vi "Wizard_Msg.vi"(0 "Application_Directory":path, 11 "Error_In":errorcluster) -> (15 "Error_Out":errorcluster)   [LabVIEW 2023]
doc: "This is a VI work as one of the front panel of the Game, showing the message of wizard."
uses:
  Controls/Bool_Button.ctl
  Controls/State.ctl
panel:
  in  "Back?":T1
  in  "Next":T1
  out "Wizard_Msg":string
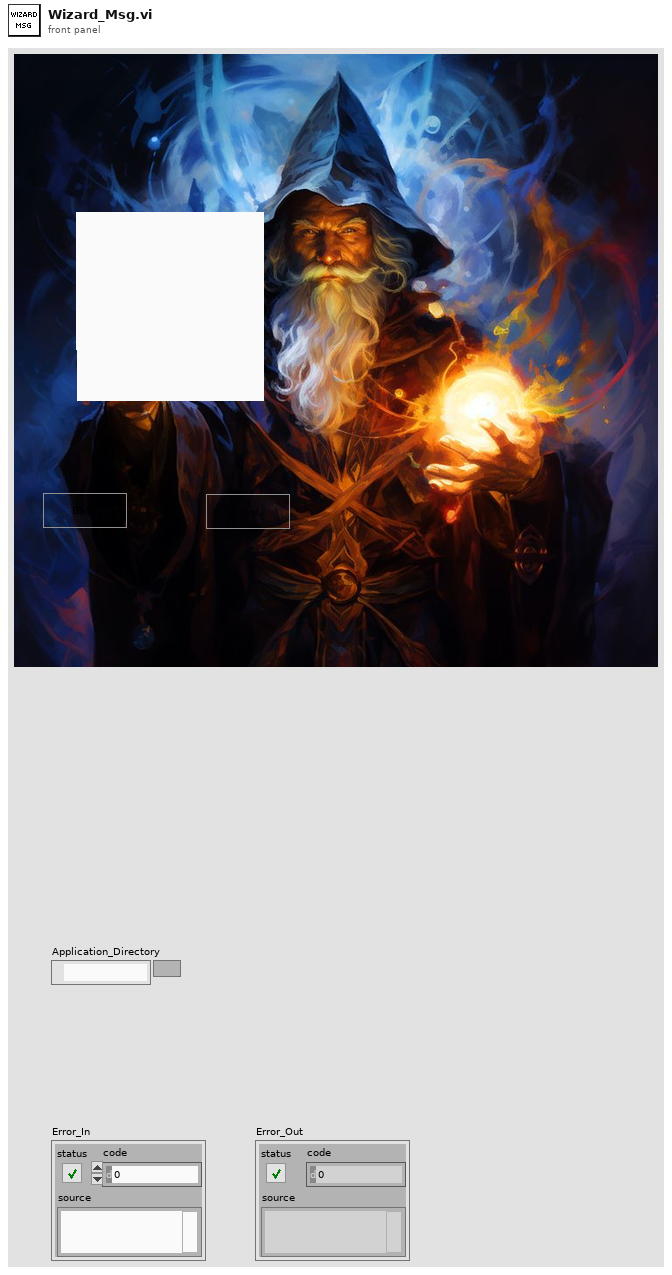
[diagram p1: front panel]
types:
  T1 = typedef "Bool_Button.ctl" = bool
  T2 = enum32{"Invalid", "Standard", "Closed", "Hidden", "Minimized", "Maximized"}
  T3 = typedef "State.ctl" = enum16{"Close", "Password_Popup", "Start_Popup", "Wizard_Msg", "Get_Name_DoB", "Lucky_Number", "Q-1", "Q-2", "Q-3", "Nature_of_the_Person"}
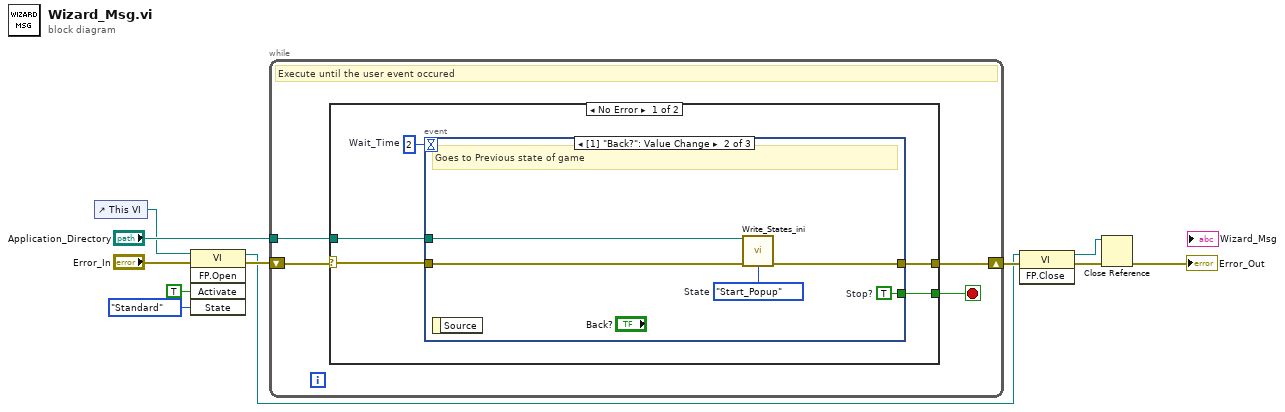
[diagram p0: block diagram]
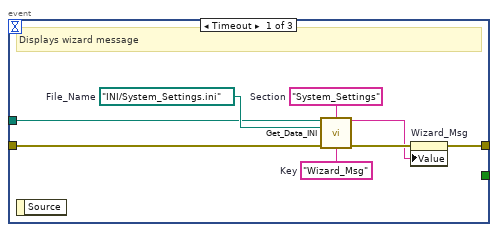
[diagram p2: hidden frame]
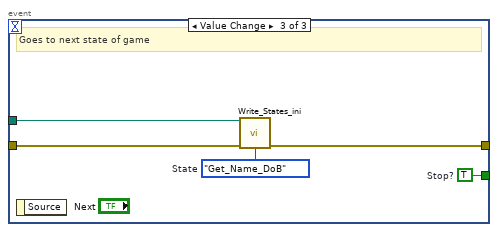
[diagram p3: hidden frame]
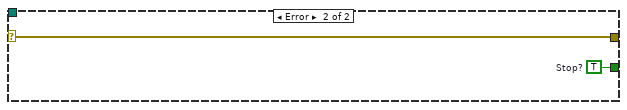
[diagram p4: hidden frame]
diagram:
  n1 = control-ref of="This VI"() -> (w8:refnum<vi>)
  n2 = invoke class="VI" method="FP.Open"(reference=w8, error in="Error_In", "Activate"=TRUE ("Activate?"), "State"=T2."Standard") -> (reference out=w1:refnum<vi>, error out=w9:errorcluster)  [unwired: 1 in, 3 out]
  n3 = while {
    tunnel: "Application_Directory" -> [w13]
    shift-right: [w14] -> w3
    shift-left: w9 -> [w15]
    stop <- w12 stop-if-true
    # "Execute until the user event occured"
    n4 = case shown="No Error" w15 {
      selector: w15 -> [w20 w40]
      tunnel: [w19 w40] -> w14
      tunnel: w13 -> [w18 _]
      tunnel: [w16 w39] -> w12
      frame No Error {
        w17 = 2  # Wait_Time
        n5 = event shown="[1] \"Back?\": Value Change" {
          selector: _ -> [_ _ _]
          dyn-events: _ -> [_ _ _]
          timeout: w17 -> [_ _ _]
          tunnel: w20 -> [w25 w30 w37]
          tunnel: [w22 w31 w36] -> w19
          tunnel: w18 -> [w24 w29 w34]
          tunnel: [_ w33 w38] -> w16
          event Timeout {
            w27 = path "INI/System_Settings.ini"  # File_Name
            w28 = "Wizard_Msg"  # Key
            w26 = "System_Settings"  # Section
            # "Displays wizard message"
            n6 = event-data() -> ()  [unwired: 1 in, 1 out]
            n7 = call "Get_Data_INI.vi"("Application_Directory"=w24, "Section"=w26, "File_Name"=w27, "Error_In"=w25, "Key"=w28) -> ("Data"=w21:string, "Error_Out"=w23:errorcluster)  [unwired: 9 in]
            n8 = property on="Wizard_Msg" class="Str"(error in=w23, "Value"=w21) -> (error out=w22:errorcluster)  [unwired: 1 in, 1 out]
          }
          event Value Change {
            w32 = State."Start_Popup"  # State
            w33 = TRUE  # Stop?
            # "Goes to Previous state of game"
            n9 = event-data() -> ()  [unwired: 1 in, 1 out]
            n10 = call "Write_States_ini.vi"("Application_Directory"=w29, "Error_In"=w30, "State"=w32) -> ("Error_Out"=w31:errorcluster)  [unwired: 12 in]
          }
          event Value Change {
            w35 = State."Get_Name_DoB"  # State
            w38 = TRUE  # Stop?
            # "Goes to next state of game"
            n11 = event-data() -> ()  [unwired: 1 in, 1 out]
            n12 = call "Write_States_ini.vi"("Application_Directory"=w34, "Error_In"=w37, "State"=w35) -> ("Error_Out"=w36:errorcluster)  [unwired: 12 in]
          }
        }
      }
      frame Error {
        w39 = TRUE  # Stop?
      }
    }
  }
  n13 = invoke class="VI" method="FP.Close"(reference=w1, error in=w3) -> (reference out=w5:refnum<vi>, error out=w4:errorcluster)  [unwired: 1 in, 1 out]
  n14 = Close Reference(reference=w5, error in (no error)=w4) -> (error out=→"Error_Out":errorcluster)
